vi "Do Action.vi"(8 "error in (no error)":errorcluster, 11 "Wait On Assert ID in":refnum<class "Wait On Assert ID.lvclass">) -> (0 "error out":errorcluster, 2 "Service out":refnum<class "Service Action Base.lvclass">)   [LabVIEW 2016, in "Assert API Components.lvlib" / "Assert Service.lvlib" / "Wait On Assert ID.lvclass"]
uses:
  Wait On Assert ID.lvclass
  D:/Work/Projects/actor_assert_api/Core/Assert Service/Service Actions/Service Action Base.lvclass
  Service Action Base.lvclass
  <vilib>/NI/STM/UDP/UDP Data Info.ctl
  <vilib>/NI/STM/SubVIs/MetaDataElement.ctl
  Wait On Assert ID.lvclass/Wait On Assert ID.ctl
  <vilib>/NI/STM/UDP/Write Message (UDP).vi
  <vilib>/NI/STM/UDP/Read Message (UDP).vi
  <vilib>/NI/STM/NI STM.lvlib
panel:
  out "data string":string
  out "name":T1
  out "data info":T2
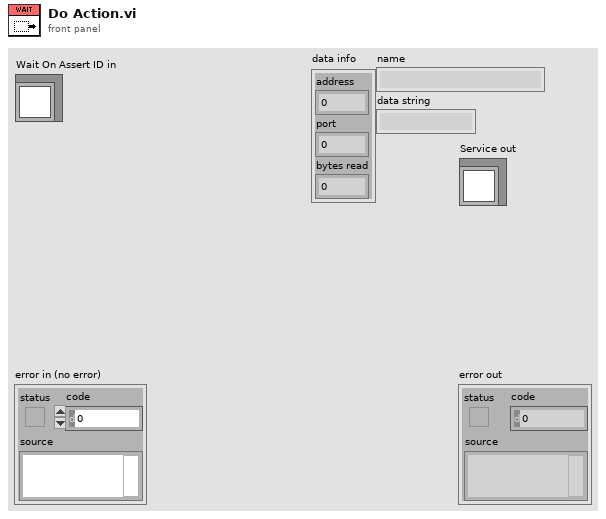
[diagram p1: front panel]
types:
  T1 = typedef "NI STM.lvlib/MetaDataElement.ctl" = string
  T2 = typedef "NI STM.lvlib/UDP Data Info.ctl" = cluster{"address":u32, "port":u16, "bytes read":i32}
  T3 = typedef "NI STM.lvlib/UDP Connection Info.ctl" = cluster{"connection ID":refnum<k16>, "meta data":T1[]}
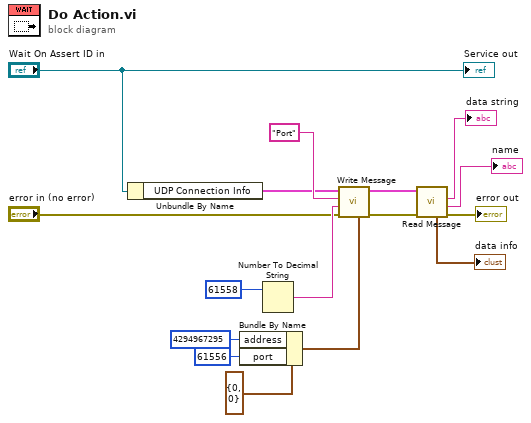
[diagram p0: block diagram]
diagram:
  n1 = Unbundle By Name("Wait On Assert ID in") -> ("UDP Connection Info"=w8:T3)
  n2 = Bundle By Name(cluster=cluster{"address":u32, "port":u16} {"address"=0, "port"=0} ("address"), "address"=u32 4294967295, "port"=u16 61556) -> (w1:cluster{"address":u32, "port":u16})
  n3 = Number To Decimal String(number=u16 61558 ("port")) -> (decimal integer string=w9:string)  [unwired: 1 in]
  n4 = call-poly <vilib>:"Write Message.vi"("address"=w1, "error in"="error in (no error)", "data"=w9, "name"="Port", "connection info in"=w8) -> ("error out"=w5:errorcluster, "connection info out"=w6:T3)  [unwired: 5 in]
  n5 = call-poly <vilib>:"Read Message.vi"("error in"=w5, "connection info in"=w6) -> ("error out"=→"error out":errorcluster, "name"=→"name":T1, "data string"=→"data string":string, "data info"=→"data info":T2)  [unwired: 4 in, 2 out]
  "Service out" <- "Wait On Assert ID in"
